vi "ShipmentClarity.vi"(6 "产品种类":u16(ring) items=["外购带卡", "外购不带卡", "自产"], 7 "包装箱条码":string, 8 "error in":errorcluster caption="错误输入", 9 "Debug":bool, 10 "箱条码":refnum<vi>, 11 "种类":refnum<vi>) -> (0 "error out":errorcluster caption="错误输出", 1 "SNStr":string, 2 "包装方式":u32, 3 "外购？":bool)   [LabVIEW 2013]
panel:
  out "ArrayOut":string[](array[string])
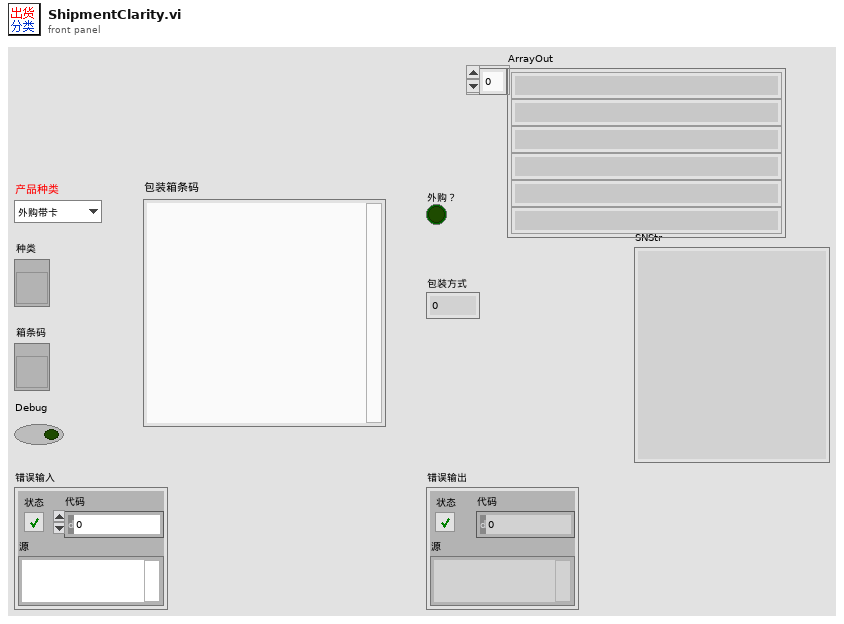
[diagram p1: front panel]
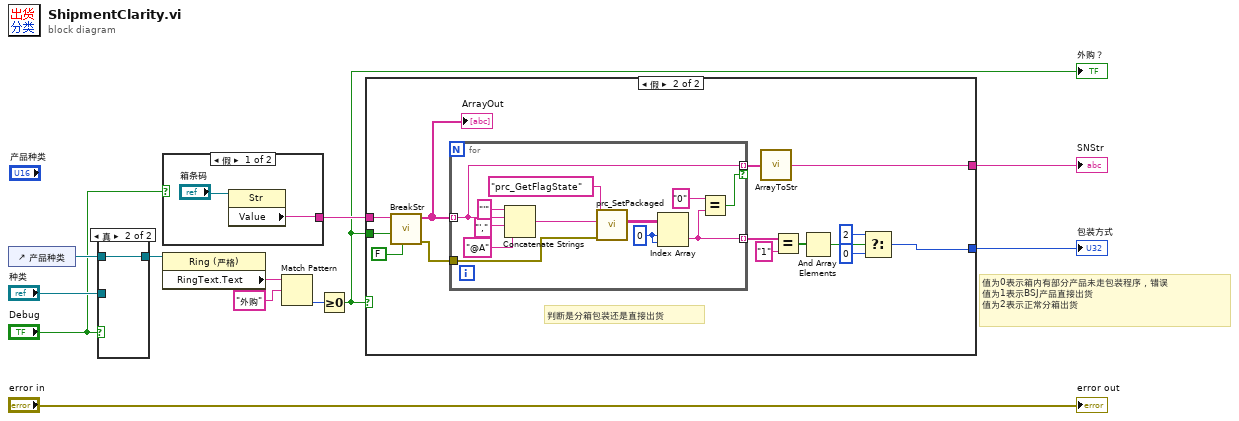
[diagram p0: block diagram]
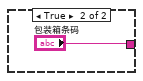
[diagram p2: hidden frame]
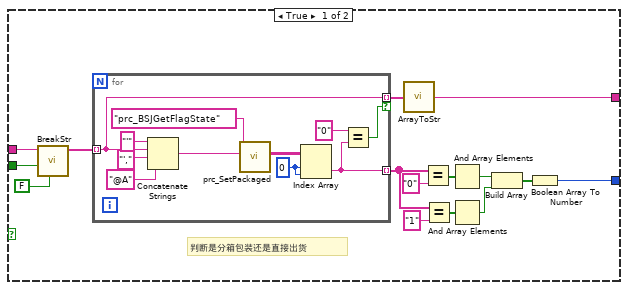
[diagram p3: hidden frame]
diagram:
  # "值为0表示箱内有部分产品未走包装程序，错误\n值为1表示BSJ产品直接出货\n值为2表示正常分箱出货"
  n1 = control-ref of="产品种类"() -> (w12:refnum<vi>)
  n2 = case shown="真" "Debug" {
    tunnel: w12 -> [_ w14]
    tunnel: "种类" -> [w13 _]
    tunnel: [w13 w14] -> w10
    frame False {
    }
    frame True {
    }
  }
  n3 = case shown="假" "Debug" {
    tunnel: [w15 "包装箱条码"] -> w5
    frame False {
      n4 = property class="Str"(reference="箱条码") -> ("Value"=w15:string)  [unwired: 1 in, 2 out]
    }
    frame True {
    }
  }
  n5 = property class="Ring (严格)"(reference=w10) -> ("RingText.Text"=w9:string)  [unwired: 1 in, 2 out]
  n6 = Match Pattern(string=w9, regular expression="外购" ("正则表达式")) -> (offset past match=w7:i32)  [unwired: 1 in, 3 out]
  n7 = Greater Or Equal To 0?(x=w7) -> (x >= 0?=w1:bool)
  "外购？" <- w1
  n8 = case shown="假" w1 {
    tunnel: w5 -> [w32 w48]
    tunnel: [w21 w49] -> w3
    tunnel: [w20 w53] -> w2
    tunnel: w1 -> [w19 w45]
    frame True {
      # "判断是分箱包装还是直接出货"
      n9 = call "BreakStr.vi"("Debug?"=FALSE, "外购？"=w19, "StrIn"=w32) -> ("ArrayOut"=w31:string[])  [unwired: 7 in, 1 out]
      n10 = for {
        tunnel: w31 -> [w36] mode=indexing
        tunnel: [w35] -> w28 mode=indexing
        tunnel: [w36] -> w23 mode=indexing if=w33
        w37 = 0
        n11 = Concatenate Strings("'", w36, "',", "@A" ("字符串")) -> (w39:string)
        n12 = call "prc_SetPackaged.vi"("string"=w39, "SQL query"="prc_BSJGetFlagState") -> ("Array"=w38:string[][])  [unwired: 8 in, 1 out]
        n13 = Index Array(array=w38, index (row)=w37, index (col)=w37) -> (element=w35:string)
        n14 = Equal?(x="0", y=w35) -> (x = y?=w33:bool)
      }
      n15 = call "ArrayToStr.vi"("Array"=w23) -> ("Str"=w20:string)
      n16 = Equal?(x=w28, y="0") -> (x = y?=w27:bool[])
      n17 = Equal?(x=w28, y="1") -> (x = y?=w26:bool[])
      n18 = And Array Elements(Boolean array=w27) -> (logical AND=w25:bool)
      n19 = And Array Elements(Boolean array=w26) -> (logical AND=w24:bool)
      n20 = Build Array(w25, w24) -> (w22:bool[])
      n21 = Boolean Array To Number(Boolean array=w22) -> (number=w21:u32)
    }
    frame False {
      # "判断是分箱包装还是直接出货"
      n22 = call "BreakStr.vi"("Debug?"=FALSE, "外购？"=w45, "StrIn"=w48) -> ("error out"=w46:errorcluster, "ArrayOut"=w47:string[])  [unwired: 7 in]
      "ArrayOut" <- w47
      n23 = for {
        tunnel: w47 -> [w62] mode=indexing
        tunnel: [w61] -> w56 mode=indexing
        tunnel: [w62] -> w54 mode=indexing if=w59
        tunnel: w46 -> [w58]
        w63 = 0
        n24 = Concatenate Strings("'", w62, "',", "@A" ("字符串")) -> (w65:string)
        n25 = call "prc_SetPackaged.vi"("error in"=w58, "string"=w65, "SQL query"="prc_GetFlagState") -> ("Array"=w64:string[][])  [unwired: 7 in, 1 out]
        n26 = Index Array(array=w64, index (row)=w63, index (col)=w63) -> (element=w61:string)
        n27 = Equal?(x="0", y=w61) -> (x = y?=w59:bool)
      }
      n28 = call "ArrayToStr.vi"("Array"=w54) -> ("Str"=w53:string)
      n29 = Equal?(x=w56, y="1") -> (x = y?=w55:bool[])
      n30 = And Array Elements(Boolean array=w55) -> (logical AND=w52:bool)
      n31 = Select(t=2, s=w52, f=0) -> (s? t:f=w49:i32)
    }
  }
  "包装方式" <- w3
  "SNStr" <- w2
  "error out" <- "error in"
